vi "AV Write Array.vi"(8 "error in":errorcluster, 10 "Voltage AV":dbl[](array[numeric]), 11 "Voltage Actual Value in":refnum<class "Voltage Actual Value.lvclass">) -> (0 "error out":errorcluster, 3 "Voltage Actual Value out":refnum<class "Voltage Actual Value.lvclass">)   [LabVIEW 2023, in "Voltage Actual Value.lvclass"]
uses:
  Voltage Actual Value.lvclass
  Voltage Actual Value.lvclass/Voltage Actual Value.ctl
  Parents/Actual Value/Actual Value.lvclass
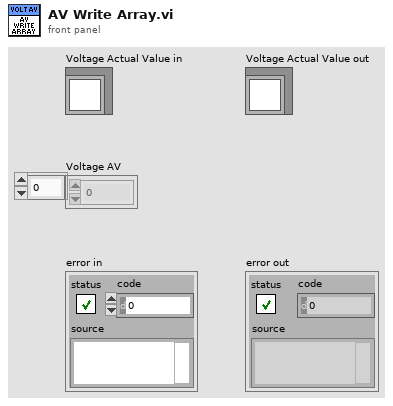
[diagram p1: front panel]
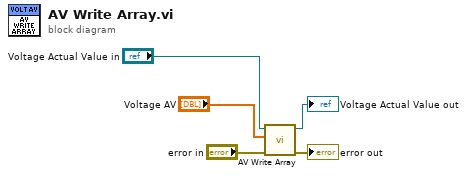
[diagram p0: block diagram]
diagram:
  n1 = call-parent "AV Write Array.vi"("error in"="error in", "Actual Value"="Voltage AV", "Actual Value in"="Voltage Actual Value in") -> ("error out"=→"error out":errorcluster, "Actual Value out"=→"Voltage Actual Value out":refnum<class "Voltage Actual Value.lvclass">)  [unwired: 7 in]
